vi "system serialize test.vi"() -> ()   [LabVIEW 2013, in "configuration tests.lvlib"]
uses:
  configuration tests.lvlib
  Framework Configuration Classes/platypus configuration/targets cluster.ctl
  Framework Configuration Classes/target configuration/PL_Target Configuration.lvclass
  Framework Configuration Classes/platypus configuration/engines cluster.ctl
  <vilib>/NI/Module Execution Interface/Engine Configuration/engine configuration.lvclass
  <vilib>/NI/Tag Bus Module Framework/module configuration/TBM module configuration.lvclass
  Framework Configuration Classes/platypus configuration/systems cluster.ctl
  Framework Configuration Classes/system configuration/PL_System Configuration.lvclass
  <vilib>/NI/Configuration Framework/serializable configuration/NISE_CEF_serializable configuration.lvclass/NISE_CEF_serializable configuration.ctl
  <vilib>/NI/Configuration Framework/serializable configuration/NISE_CEF_serializable configuration.lvclass
  Framework Configuration Classes/system configuration/PL_System Configuration.lvclass/PL_System Configuration.ctl
  Framework Configuration Classes/target configuration/PL_Target Configuration.lvclass/PL_Target Configuration.ctl
  test module/module/configuration/TEST CONFIGURATION.lvclass
  <vilib>/NI/Tag Bus/tag/Data Type.ctl
  <vilib>/NI/Tag Bus/tag/tag descriptor.lvclass
  <vilib>/NI/Tag Bus/tag/tag descriptor.lvclass/tag descriptor.ctl
  <vilib>/NI/Tag Bus/tag/read tag name.vi
  Framework Configuration Classes/target configuration/Write name.vi
  Framework Configuration Classes/system configuration/Write Configuration Name.vi
  Framework Configuration Classes/system configuration/Write save time.vi
  Framework Configuration Classes/system configuration/Read Configuration Name.vi
  Framework Configuration Classes/system configuration/Read save time.vi
  Framework Configuration Classes/target configuration/Read name.vi
  Framework Configuration Classes/platypus configuration/PLConfigurationSerializer.lvlib
panel:
  in  "tags":i32=5
  in  "modules":i32=1000
  out "desertime":dbl
  out "sertime":dbl
  out "moduleok":bool
  out "engok":bool
  out "engclasserr":errorcluster
  out "targok":bool
  out "sysok":bool
  out "sererr":errorcluster
  out "desererr":errorcluster
  out "data":string
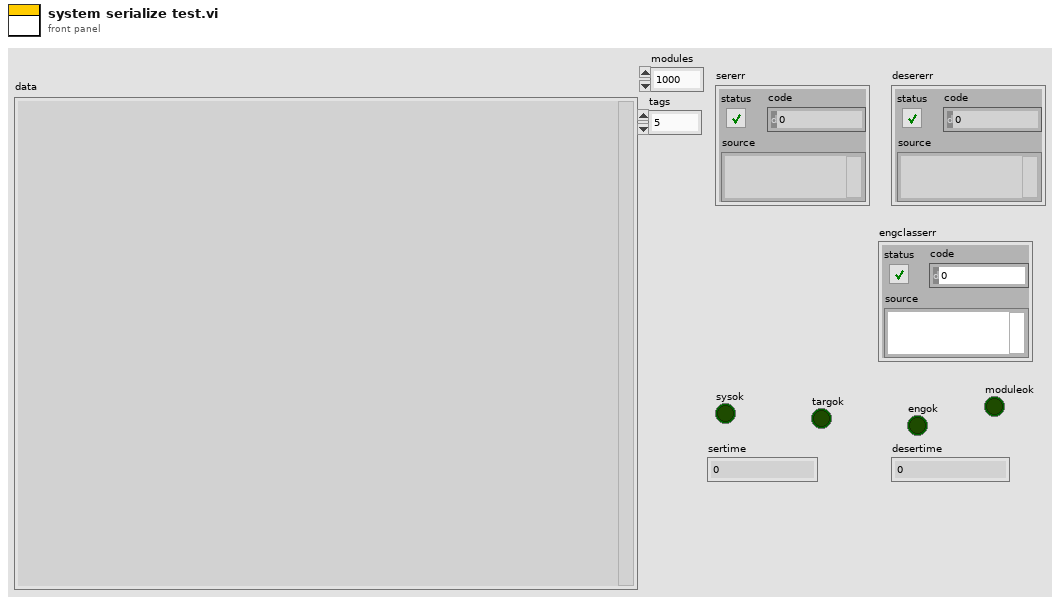
[diagram p1: front panel]
types:
  T1 = typedef "PLConfigurationSerializer.lvlib/engines cluster.ctl" = cluster{"engine configuration":refnum<class "engine configuration.lvclass">, "modules":refnum<class "TBM module configuration.lvclass">[]}
  T2 = typedef "PLConfigurationSerializer.lvlib/systems cluster.ctl" = cluster{"System Configuration":refnum<class "PL_System Configuration.lvclass">, "targets":T3[]}
  T3 = typedef "PLConfigurationSerializer.lvlib/targets cluster.ctl" = cluster{"Target Configuration":refnum<class "PL_Target Configuration.lvclass">, "engines":T1[]}
  T4 = typedef "tag bus.lvlib/tag descriptor.lvclass/Data Type.ctl" = enum16{"Double", "Single", "I64", "I32", "I16", "I8", "U64", "U32", "U16", "U8", "Boolean", "String", "Array of Double", "Array of Single", "Array of I64", "Array of I32", "Array of I16", "Array of I8", "Array of U64", "Array of U32", "Array of U16", "Array of U8", "Array of Boolean", "Array of String"}
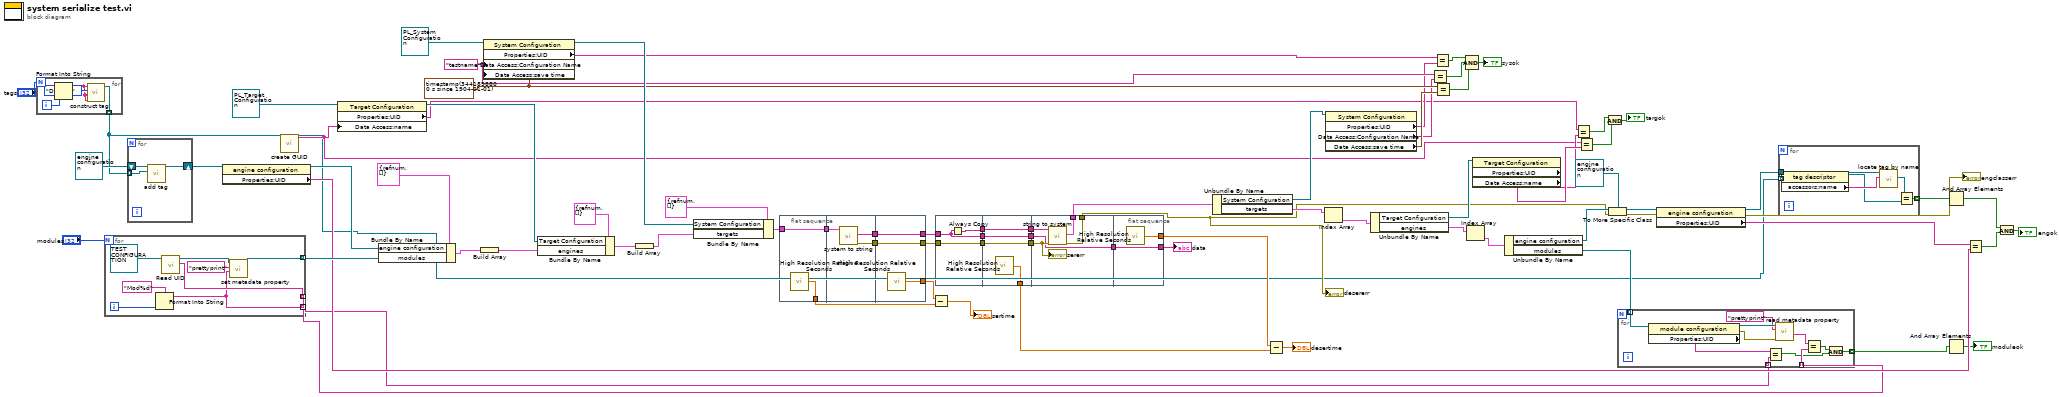
[diagram p0: block diagram]
diagram:
  w58 = timestamp(3441898800 s since 1904-01-01) ("save time")
  w59 = "testname" ("Configuration Name")
  n1 = for {
    N: "tags" -> [_]
    tunnel: [w81] -> w13 mode=indexing
    i -> [w84]
    n2 = Format Into String(w84) -> (resulting string=w82:string)  [unwired: 3 in, 1 out]
    n3 = call <vilib>:"construct tag.vi"("raw default"=w82, "metadata"=w82, "data type"=Data_Type."Double", "name"=w82) -> ("system tag out"=w81:refnum<class "tag descriptor.lvclass">)  [unwired: 6 in, 1 out]
  }
  n4 = for {
    N: "modules" -> [_]
    tunnel: [w89] -> w72 mode=indexing
    tunnel: [w87] -> w31 mode=indexing
    tunnel: [w86] -> w32 mode=indexing
    i -> [w92]
    n5 = Format Into String(format string="Mod%d", w92) -> (resulting string=w86:string)  [unwired: 2 in, 1 out]
    n6 = call <vilib>:"Read UID.vi"("configuration in"=refnum<class "TEST CONFIGURATION.lvclass"> refnum ("configuration tests.lvlib:user module configuration")) -> ("instance id"=w87:string, "configuration out"=w90:refnum<class "TEST CONFIGURATION.lvclass">)  [unwired: 8 in, 1 out]
    n7 = call <vilib>:"set metadata property.vi"("value"=w86, "key"="prettyprint", "configuration in"=w90) -> ("configuration out"=w89:refnum<class "TEST CONFIGURATION.lvclass">)  [unwired: 7 in, 1 out]
  }
  n8 = for {
    shift-right: [w94] -> w15
    shift-left: refnum<class "engine configuration.lvclass"> refnum ("Engine Configuration") -> [w95]
    tunnel: w13 -> [w93] mode=indexing
    n9 = call <vilib>:"add tag.vi"("tag descriptor"=w93, "engine configuration in"=w95) -> ("engine configuration out"=w94:refnum<class "engine configuration.lvclass">)  [unwired: 8 in, 1 out]
  }
  n10 = property class="engine configuration"(reference=w15) -> (reference out=w71:refnum<class "engine configuration.lvclass">, "Properties:UID"=w34:string)  [unwired: 1 in, 1 out]
  n11 = call <vilib>:"create GUID.vi"() -> ("uuid"=w44:string)  [unwired: 11 in]
  n12 = property class="Target Configuration"(reference=refnum<class "PL_Target Configuration.lvclass"> refnum ("Target Configuration"), "Data Access:name"=w44) -> (reference out=w69:refnum<class "PL_Target Configuration.lvclass">, "Properties:UID"=w43:string)  [unwired: 1 in, 1 out]
  n13 = Bundle By Name(cluster=T1 {"engine configuration"=refnum, "modules"=[]} ("engines cluster"), "engine configuration"=w71, "modules"=w72) -> (w79:T1)
  n14 = Build Array(w79) -> (w77:T1[])
  n15 = property class="System Configuration"(reference=refnum<class "PL_System Configuration.lvclass"> refnum ("System Configuration"), "Data Access:Configuration Name"=w59, "Data Access:save time"=w58) -> (reference out=w67:refnum<class "PL_System Configuration.lvclass">, "Properties:UID"=w60:string)  [unwired: 1 in, 1 out]
  n16 = Bundle By Name(cluster=T3 {"Target Configuration"=refnum, "engines"=[]} ("targets cluster"), "Target Configuration"=w69, "engines"=w77) -> (w76:T3)
  n17 = Build Array(w76) -> (w74:T3[])
  n18 = Bundle By Name(cluster=T2 {"System Configuration"=refnum, "targets"=[]} ("system"), "System Configuration"=w67, "targets"=w74) -> (w20:T2)
  n19 = flat-sequence {
    tunnel: w20 -> [w97]
    tunnel: [w97] -> w26
    tunnel: [w96] -> w24
    tunnel: [w100] -> w27
    tunnel: w26 -> [w99]
    tunnel: [w98] -> w8
    tunnel: [w103] -> w73
    tunnel: w27 -> [w103]
    tunnel: [w102] -> w25
    tunnel: [w101] -> w9
    tunnel: w8 -> [w101]
    frame #0 {
      n20 = call <vilib>:"High Resolution Relative Seconds.vi"() -> ("relative seconds"=w96:dbl)
    }
    frame #1 {
      n21 = call "system to string.vi"("system"=w99) -> ("error out"=w100:errorcluster, "data"=w98:string)  [unwired: 9 in]
    }
    frame #2 {
      n22 = call <vilib>:"High Resolution Relative Seconds.vi"() -> ("relative seconds"=w102:dbl)
    }
  }
  n23 = Subtract(x=w25, y=w24) -> (x-y=→"sertime":dbl)
  n24 = flat-sequence {
    tunnel: w9 -> [w104]
    tunnel: w73 -> [w106]
    tunnel: [w106] -> w7
    tunnel: [w105] -> w6
    tunnel: [w104] -> w5
    tunnel: [w110] -> w28
    tunnel: [w109] -> w21
    tunnel: [w108] -> w10
    tunnel: w7 -> [w110]
    tunnel: w6 -> [w108]
    tunnel: w5 -> [w107]
    tunnel: [w107] -> w4
    tunnel: [w114] -> w19
    tunnel: [w113] -> w40
    tunnel: w28 -> [w115]
    tunnel: w10 -> [w112]
    tunnel: w4 -> [w111]
    tunnel: [w111] -> w3
    tunnel: [w117] -> w22
    tunnel: [w116] -> w2
    tunnel: w3 -> [w116]
    frame #0 {
      n25 = Always Copy(1:w104) -> (0:w105:string)
    }
    frame #1 {
      n26 = call <vilib>:"High Resolution Relative Seconds.vi"() -> ("relative seconds"=w109:dbl)
    }
    frame #2 {
      n27 = call "string to system.vi"("error in"=w115, "data"=w112) -> ("error out"=w113:errorcluster, "system"=w114:T2)  [unwired: 8 in]
      "sererr" <- w115
    }
    frame #3 {
      n28 = call <vilib>:"High Resolution Relative Seconds.vi"() -> ("relative seconds"=w117:dbl)
    }
  }
  n29 = Unbundle By Name(w19) -> ("System Configuration"=w61:refnum<class "PL_System Configuration.lvclass">, "targets"=w65:T3[])
  n30 = Subtract(x=w22, y=w21) -> (x-y=→"desertime":dbl)
  n31 = Index Array(array=w65) -> (element=w63:T3)  [unwired: 1 in]
  n32 = property class="System Configuration"(reference=w61) -> ("Properties:UID"=w55:string, "Data Access:Configuration Name"=w56:string, "Data Access:save time"=w57:timestamp)  [unwired: 1 in, 2 out]
  n33 = Unbundle By Name(w63) -> ("Target Configuration"=w50:refnum<class "PL_Target Configuration.lvclass">, "engines"=w64:T1[])
  n34 = Equal?(x=w59, y=w56) -> (x = y?=w53:bool)
  n35 = Equal?(x=w60, y=w55) -> (x = y?=w54:bool)
  n36 = Equal?(x=w58, y=w57) -> (x = y?=w52:bool)
  n37 = Compound Arithmetic op=AND(w54, w53, w52) -> (→"sysok":bool)
  n38 = Index Array(array=w64) -> (element=w62:T1)  [unwired: 1 in]
  n39 = property class="Target Configuration"(reference=w50) -> ("Properties:UID"=w45:string, "Data Access:name"=w46:string)  [unwired: 1 in, 2 out]
  n40 = Unbundle By Name(w62) -> ("engine configuration"=w42:refnum<class "engine configuration.lvclass">, "modules"=w33:refnum<class "TBM module configuration.lvclass">[])
  n41 = Equal?(x=w43, y=w45) -> (x = y?=w47:bool)
  n42 = Equal?(x=w44, y=w46) -> (x = y?=w48:bool)
  n43 = Compound Arithmetic op=AND(w47, w48) -> (→"targok":bool)
  n44 = To More Specific Class(target class=refnum<class "engine configuration.lvclass"> refnum ("Engine Configuration"), reference=w42, error in=w40) -> (specific class reference=w41:refnum<class "engine configuration.lvclass">, error out=w39:errorcluster)
  n45 = for {
    tunnel: w33 -> [w128] mode=indexing
    tunnel: w32 -> [w123] mode=indexing
    tunnel: w31 -> [w121] mode=indexing
    tunnel: [w118] -> w30 mode=indexing
    n46 = property class="module configuration"(reference=w128) -> (reference out=w127:refnum<class "TBM module configuration.lvclass">, error out=w125:errorcluster, "Properties:UID"=w122:string)  [unwired: 1 in]
    n47 = Equal?(x=w122, y=w121) -> (x = y?=w119:bool)
    n48 = call <vilib>:"read metadata property.vi"("error in"=w125, "key"="prettyprint", "configuration in"=w127) -> ("value"=w124:string)  [unwired: 5 in, 3 out]
    n49 = Equal?(x=w124, y=w123) -> (x = y?=w120:bool)
    n50 = And(x=w120, y=w119) -> (x .and. y?=w118:bool)
  }
  n51 = property class="engine configuration"(reference=w41, error in=w39) -> (reference out=w14:refnum<class "engine configuration.lvclass">, error out=→"engclasserr":errorcluster, "Properties:UID"=w35:string)
  n52 = for {
    tunnel: w14 -> [w134]
    tunnel: w13 -> [w133] mode=indexing
    tunnel: [w129] -> w12 mode=indexing
    n53 = property class="tag descriptor"(reference=w133) -> (reference out=w130:refnum<class "tag descriptor.lvclass">, "accessors:name"=w132:string)  [unwired: 1 in, 1 out]
    n54 = call <vilib>:"locate tag by name.vi"("tag name"=w132, "engine configuration in"=w134) -> ("tag descriptor"=w131:refnum<class "tag descriptor.lvclass">)  [unwired: 7 in, 2 out]
    n55 = Equal?(x=w131, y=w130) -> (x = y?=w129:bool)
  }
  n56 = And Array Elements(Boolean array=w30) -> (logical AND=→"moduleok":bool)
  n57 = And Array Elements(Boolean array=w12) -> (logical AND=w11:bool)
  n58 = Equal?(x=w35, y=w34) -> (x = y?=w37:bool)
  n59 = Compound Arithmetic op=AND(w11, w37) -> (→"engok":bool)
  "desererr" <- w40
  "data" <- w2
